vi "Measurement UI.vi"() -> ()   [LabVIEW 2021, in "Generation_Class D Amplifier_UI.lvlib"]
uses:
  Generation_Class D Amplifier_UI.lvlib
  Generation_Class D Amplifier/generation control.ctl
  shared/controls/digital output level units.ctl
  service/generation/controls/generation status.ctl
  shared/controls/generation type.ctl
  <vilib>/Utility/miscctls.llb/LVPositionTypeDef.ctl
  service/generation/controls/generation type.ctl
  service/generation/API/AudioGeneration/AudioGeneration.lvclass
  service/generation/controls/AudioGenTypeDefs.lvlib
  shared/audio popup ui/Audio Popup UI.lvlib
  Generation_Class D Amplifier/Generation_Class D Amplifier.lvlib
  shared/controls/audio controls.lvlib
panel:
  in  "configure output":bool
  in  "output type":T1 caption="Generation Type"
  in  "master clock channel list":string caption="Master Clock Channel"
  in  "digital channel list":string caption="Digital Audio Channel"
  in  "output configuration file":string
  out "wfm - data":dbl[](array[numeric])
  out "wfm - dt":dbl
  out "wfm - t0":dbl
  in  "signal phase":dbl caption="phase"
  out "status":T2 caption="Status"
  in  "signal frequency":dbl=1000.0 caption="Frequency" format="%#_6pHz"
  in  "output level":dbl=-1.0 caption="Output level" format="%#_3f"
  in  "output level units":T3
  in  "enable dither":bool caption="Enable dither"
  in  "generation control":T4=enum."Stop" caption="Action"
  # "Generation"
  # "Harware Resource"
  # "Signal Generation"
  # "hidden controls - used to sync with MeasLink"
  # "hidden indicators"
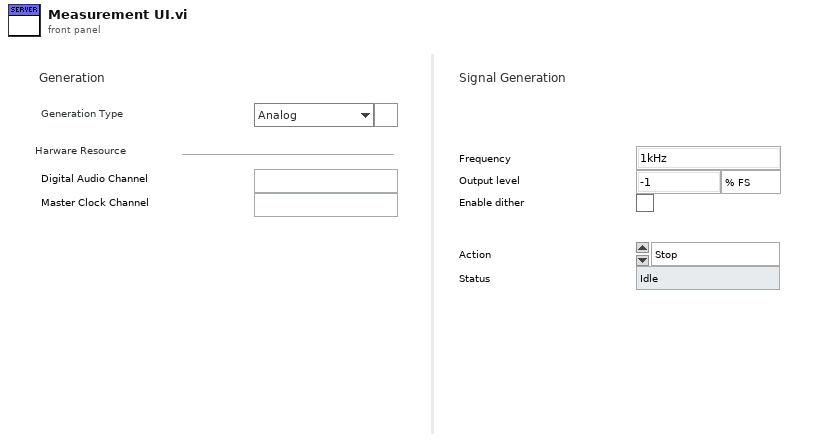
[diagram p1: front panel]
types:
  T1 = typedef "generation type.ctl" = enum32{"Analog", "Digital Serial"}
  T2 = typedef "AudioGenTypeDefs.lvlib/generation status.ctl" = enum16{"Idle", "Committed", "Active"}
  T3 = typedef "audio controls.lvlib/digital output level units.ctl" = enum32{"% FS", "dBFS"}
  T4 = typedef "Generation_Class D Amplifier.lvlib/generation control.ctl" = enum32{"Start", "Stop"}
  T5 = typedef "AudioGenTypeDefs.lvlib/generation type.ctl" = enum16{"analog", "digital"}
  T6 = typedef "LVPositionTypeDef.ctl" = cluster{"Left":i32, "Top":i32}
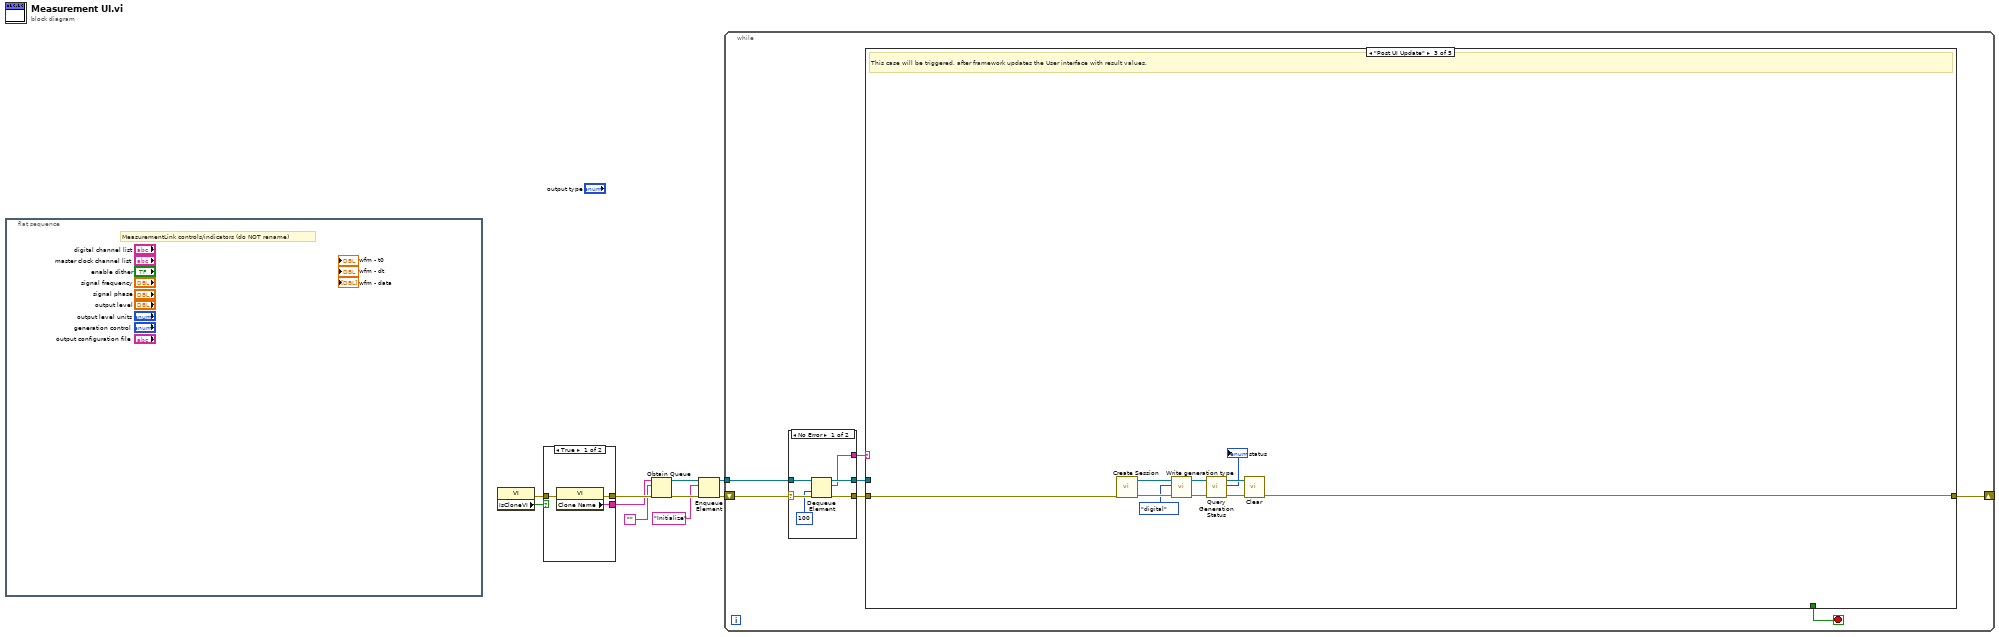
[diagram p0: block diagram]
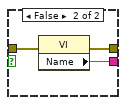
[diagram p2: hidden frame]
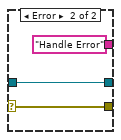
[diagram p3: hidden frame]
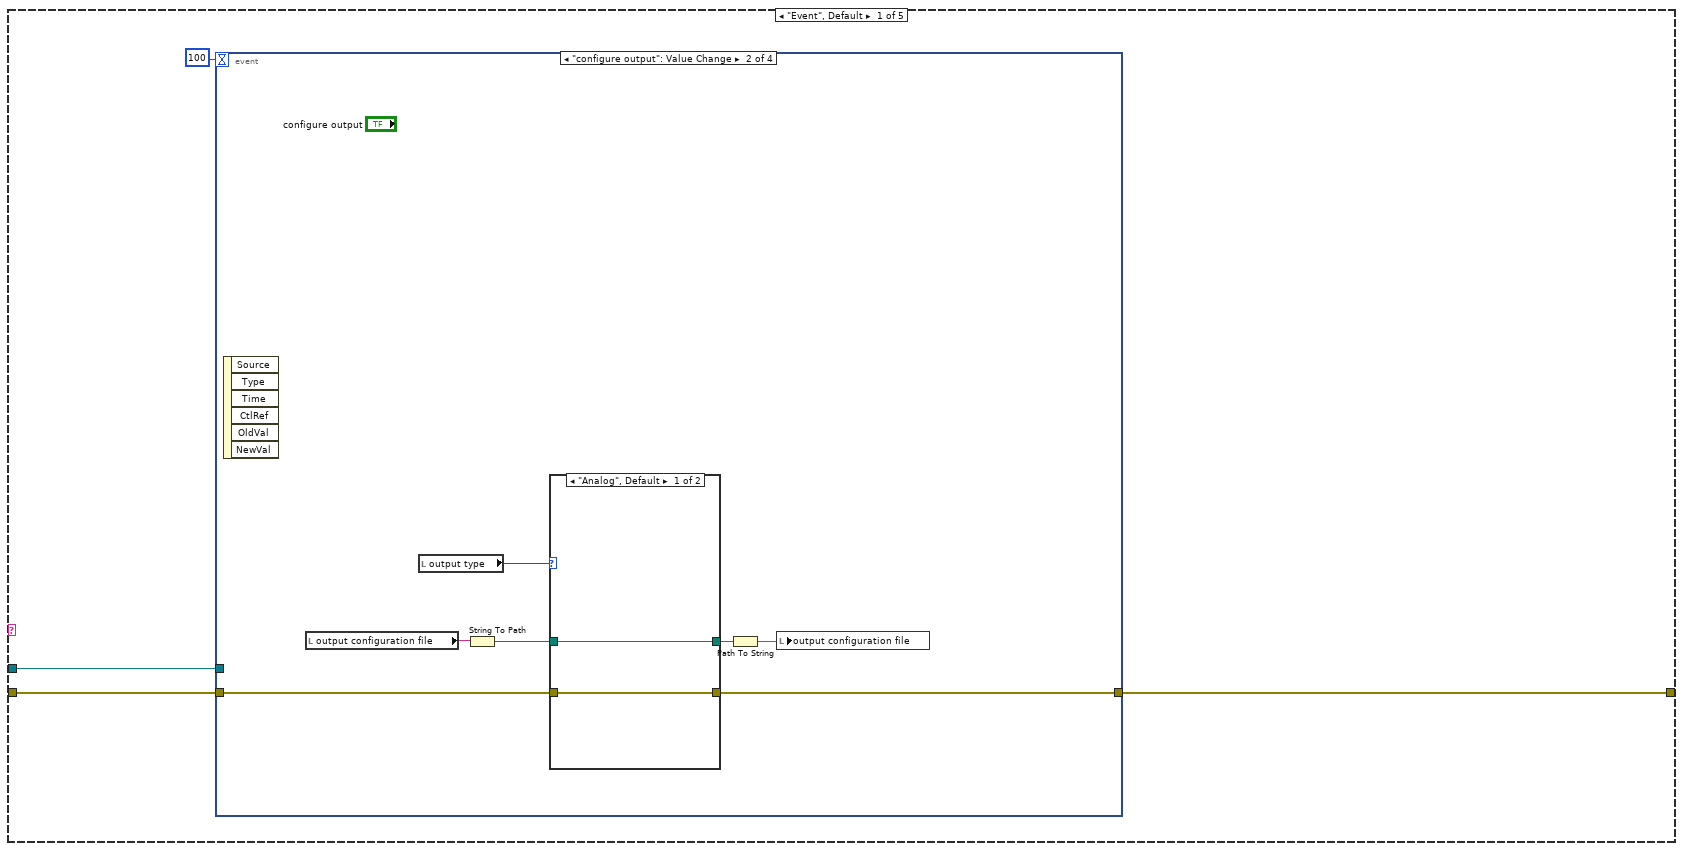
[diagram p4: hidden frame]
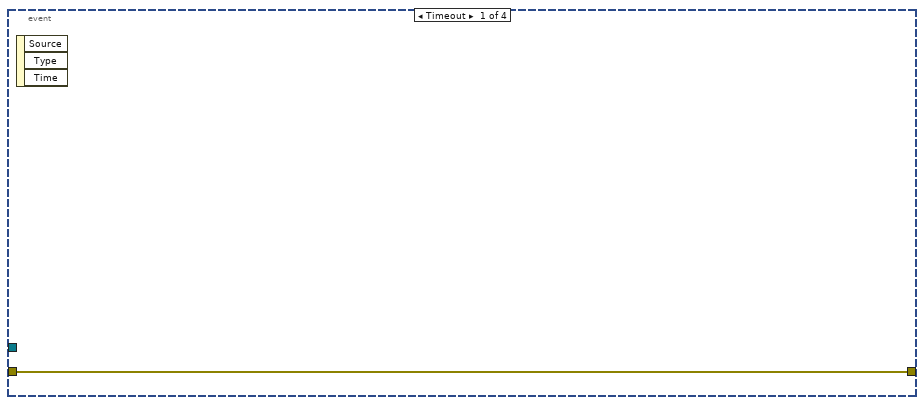
[diagram p5: hidden frame]
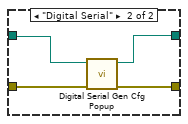
[diagram p6: hidden frame]
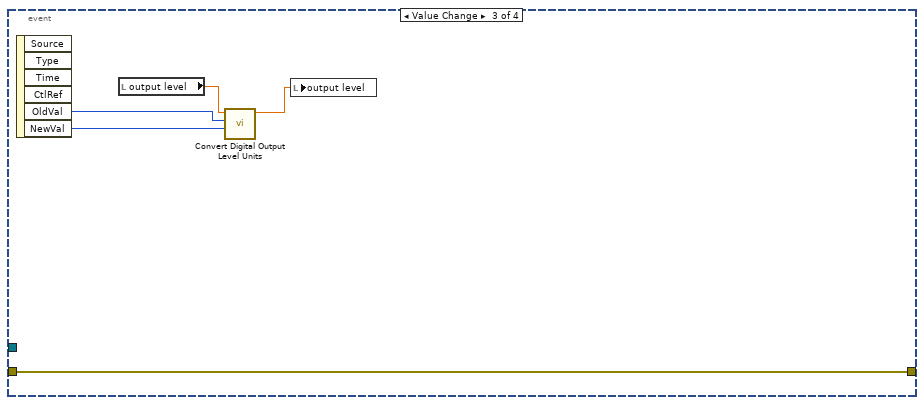
[diagram p7: hidden frame]
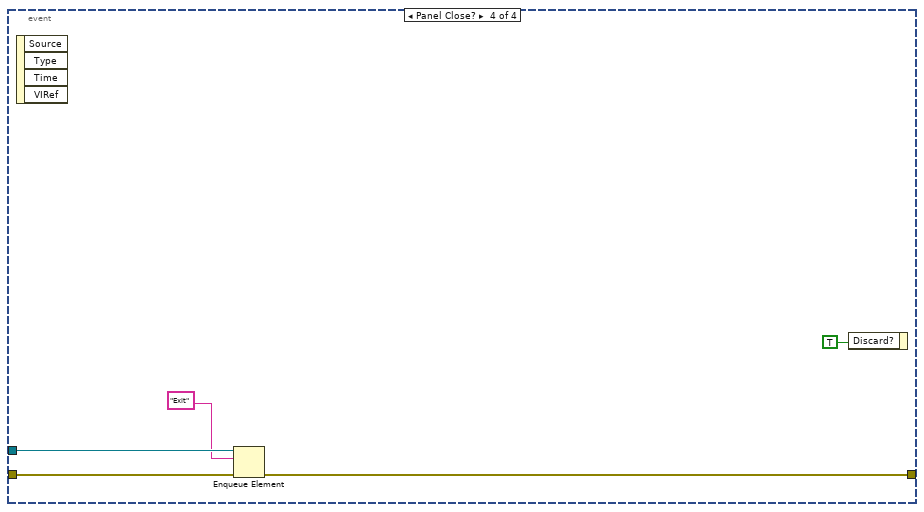
[diagram p8: hidden frame]
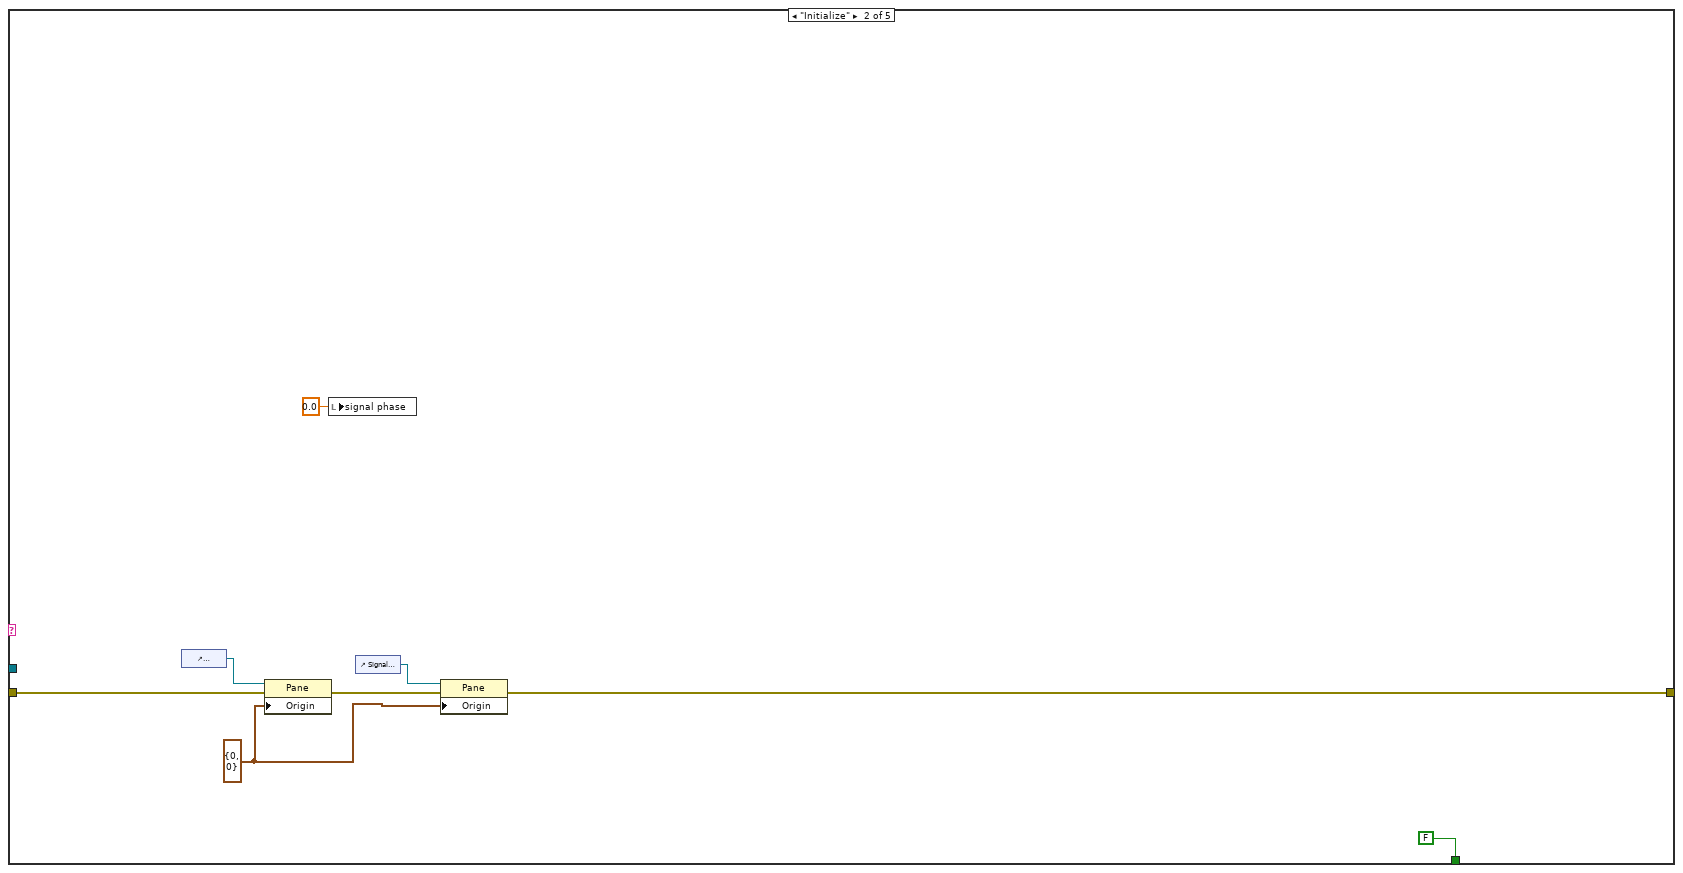
[diagram p9: hidden frame]
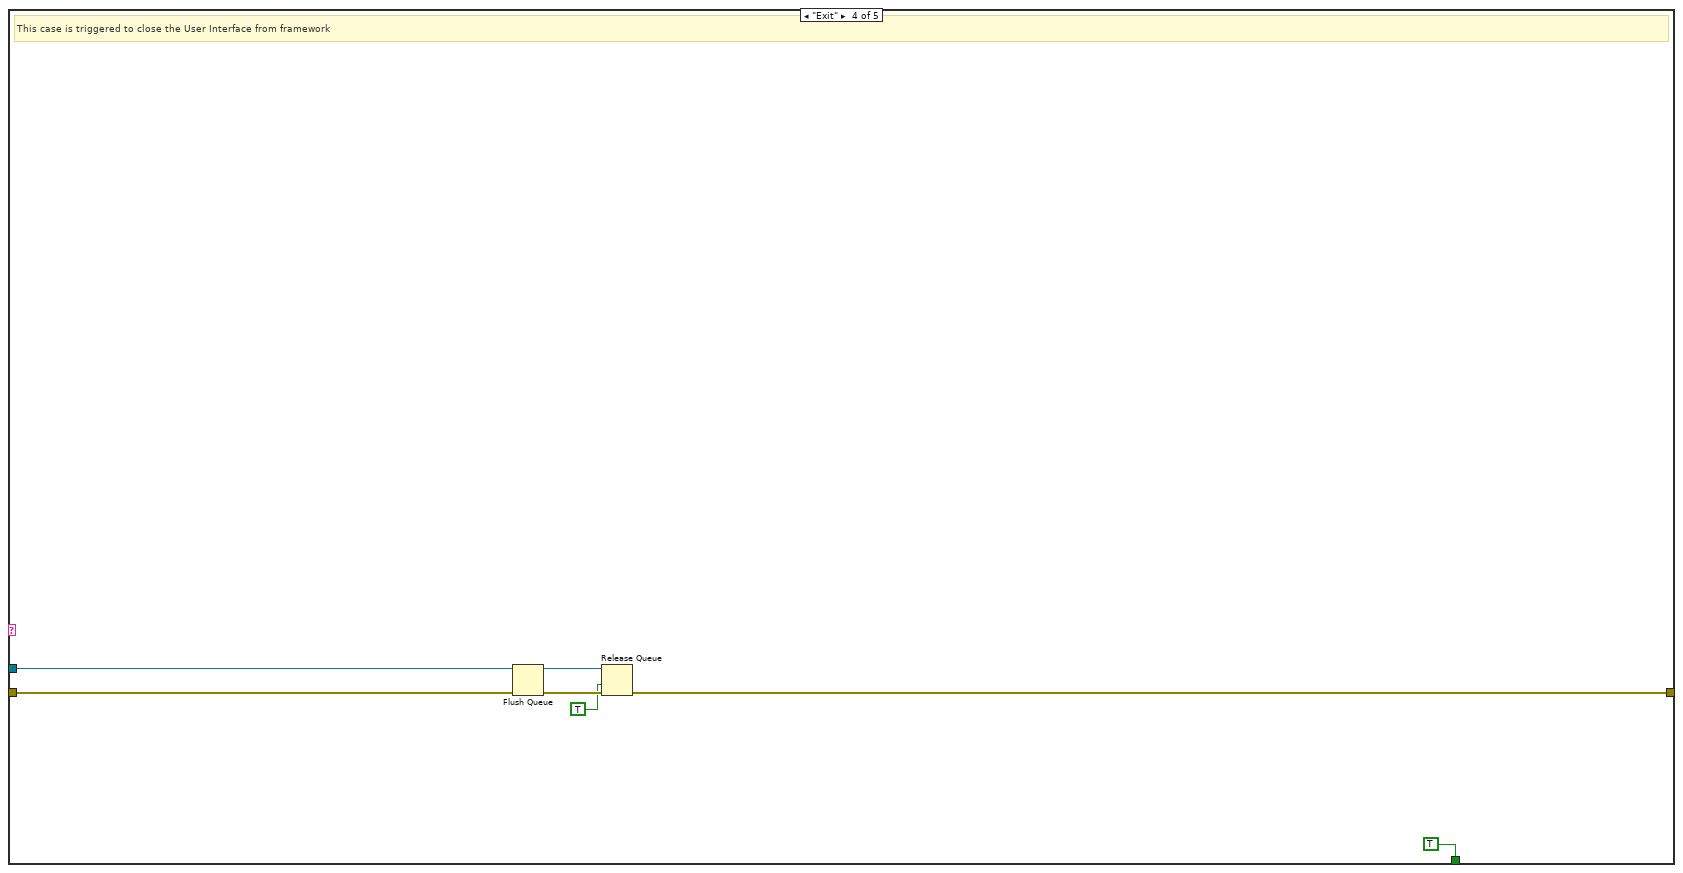
[diagram p10: hidden frame]
diagram:
  n1 = flat-sequence {
    frame #0 {
      # "MeasurementLink controls/indicators (do NOT rename)"
    }
  }
  n2 = property class="VI"() -> (error out=w1:errorcluster, "IsCloneVI"=w2:bool)  [unwired: 2 in, 1 out]
  n3 = case shown="True" w2 {
    tunnel: [w13 w16] -> w10
    tunnel: [w12 w15] -> w9
    tunnel: w1 -> [w11 w14]
    frame True {
      n4 = property class="VI"(error in=w11) -> (error out=w13:errorcluster, "Clone Name"=w12:string)  [unwired: 1 in, 1 out]
    }
    frame False {
      n5 = property class="VI"(error in=w14) -> (error out=w16:errorcluster, "Name"=w15:string)  [unwired: 1 in, 1 out]
    }
  }
  n6 = Obtain Queue(name (unnamed)=w9, element data type="", error in (no error)=w10) -> (queue out=w6:refnum<queue>, error out=w8:errorcluster)  [unwired: 2 in, 1 out]
  n7 = Enqueue Element(queue=w6, element="Initialize", error in (no error)=w8) -> (queue out=w5:refnum<queue>, error out=w7:errorcluster)  [unwired: 1 in, 1 out]
  n8 = while {
    shift-right: [w18] -> _
    shift-left: w7 -> [w23]
    tunnel: w5 -> [w21]
    stop <- w17 stop-if-true
    n9 = case shown="No Error" w23 {
      selector: w23 -> [w29 w32]
      tunnel: [w28 w32] -> w22
      tunnel: w21 -> [w27 w31]
      tunnel: [w26 w31] -> w20
      tunnel: [w25 "Handle Error"] -> w19
      frame No Error {
        n10 = Dequeue Element(queue=w27, timeout in ms (-1)=100, error in (no error)=w29) -> (queue out=w26:refnum<queue>, element=w25:string, error out=w28:errorcluster)  [unwired: 1 out]
      }
      frame Error {
      }
    }
    n11 = case shown="\"Post UI Update\"" w19 {
      tunnel: w22 -> [w35 w66 w78 w85 w86]
      tunnel: w20 -> [w33 _ _ w83 _]
      tunnel: [w36 w63 w77 w80 w86] -> w18
      tunnel: [_ FALSE _ TRUE _] -> w17
      frame "Event", Default {
        n12 = event shown="[1] \"configure output\": Value Change" {
          selector: _ -> [_ _ _ _]
          dyn-events: _ -> [_ _ _ _]
          timeout: 100 -> [_ _ _ _]
          tunnel: [w37 w43 w55 w58] -> w36
          tunnel: w35 -> [w37 w44 w55 w59]
          tunnel: w33 -> [_ _ _ w57]
          event Timeout {
            n13 = event-data() -> ()  [unwired: 1 in, 3 out]
          }
          event "configure output": Value Change {
            n14 = event-data() -> ()  [unwired: 1 in, 6 out]
            n15 = local read "output configuration file"() -> (w41:string)
            n16 = local read "output type"() -> (w42:T1)
            n17 = String To Path(string=w41) -> (path=w40:path)
            n18 = case shown="\"Analog\", Default" w42 {
              tunnel: w44 -> [w45 w50]
              tunnel: [w45 w49] -> w43
              tunnel: w40 -> [w46 w48]
              tunnel: [w46 w47] -> w39
              frame "Analog", Default {
              }
              frame "Digital Serial" {
                n19 = call "Digital Serial Gen Cfg Popup.vi"("error in (no error)"=w50, "config file in"=w48) -> ("error out"=w49:errorcluster, "config file out"=w47:path)  [unwired: 7 in, 1 out]
              }
            }
            n20 = Path To String(path=w39) -> (string=w38:string)
            n21 = local write "output configuration file"(w38) -> ()
          }
          event Value Change {
            n22 = event-data() -> ("OldVal"=w54:T3, "NewVal"=w53:T3)  [unwired: 1 in, 4 out]
            n23 = local read "output level"() -> (w52:dbl)
            n24 = call "Convert Digital Output Level Units.vi"("new output level units"=w53, "previous output level units"=w54, "previous output level"=w52) -> ("new output level"=w51:dbl)  [unwired: 8 in]
            n25 = local write "output level"(w51) -> ()
          }
          event Panel Close? {
            n26 = event-data() -> ()  [unwired: 1 in, 4 out]
            n27 = Enqueue Element(queue=w57, element="Exit", error in (no error)=w59) -> (error out=w58:errorcluster)  [unwired: 1 in, 2 out]
            n28 = event-data("Discard?"=TRUE) -> ()  [unwired: 1 in, 1 out]
          }
        }
      }
      frame "Initialize" {
        w64 = T6 {"Left"=0, "Top"=0} ("Position")
        n29 = control-ref of="OutputConfigPane"() -> (w61:refnum<vi>)
        n30 = property class="Pane"(reference=w61, error in=w66, "Origin"=w64) -> (error out=w65:errorcluster)  [unwired: 1 out]
        n31 = local write "signal phase"(0.0 ("signal phase")) -> ()
        n32 = control-ref of="Signal Generation Pane"() -> (w62:refnum<vi>)
        n33 = property class="Pane"(reference=w62, error in=w65, "Origin"=w64) -> (error out=w63:errorcluster)  [unwired: 1 out]
      }
      frame "Post UI Update" {
        # "This case will be triggered, after framework updates the User interface with result values."
        n34 = call "Create Session.vi"("error in (no error)"=w78) -> ("error out"=w75:errorcluster, "session out"=w76:refnum<class "AudioGeneration.lvclass">)  [unwired: 9 in]
        n35 = call-dynamic "Write generation type.vi"("error in (no error)"=w75, "generation type"=generation_type."digital", "AudioGeneration in"=w76) -> ("error out"=w73:errorcluster, "AudioGeneration out"=w74:refnum<class "AudioGeneration.lvclass">)  [unwired: 7 in]
        n36 = call "Query Generation Status.vi"("error in (no error)"=w73, "AudioGeneration in"=w74) -> ("error out"=w72:errorcluster, "status"=→"status":T2, "AudioGeneration out"=w71:refnum<class "AudioGeneration.lvclass">)  [unwired: 6 in, 1 out]
        n37 = call "Clear.vi"("error in (no error)"=w72, "AudioGeneration in"=w71) -> ("error out"=w77:errorcluster)  [unwired: 9 in]
      }
      frame "Exit" {
        # "This case is triggered to close the User Interface from framework"
        n38 = Flush Queue(queue=w83, error in (no error)=w85) -> (queue out=w82:refnum<queue>, error out=w81:errorcluster)  [unwired: 1 out]
        n39 = Release Queue(queue=w82, force destroy? (F)=TRUE, error in (no error)=w81) -> (error out=w80:errorcluster)  [unwired: 2 out]
      }
      frame "Handle Error" {
      }
    }
  }
